vi "DCS_positioningEvan.vi"(8 "error in (no error)":errorcluster, 9 "Data":dbl[](array[numeric])=[0.21428571428571427, 0.8571428571428571, 1.0, 0.21428571428571427, 0.9285714285714285, 0.5, 0.9285714285714285, 0.14285714285714285]) -> (0 "X-Y position":dbl[](array[numeric]), 3 "Normalized Data":dbl[][](array[numeric]))   [LabVIEW 2013]
uses:
  <vilib>/Utility/file.llb/Read From Spreadsheet File (DBL).vi
panel:
  out "Simulated array dimensions":i32[](array[numeric])
  out "output array":dbl[][](array[numeric])=[[0.21428571428571427, 0.8571428571428571, 1.0, 0.21428571428571427, 0.9285714285714285, 0.5, 0.9285714285714285, 0.14285714285714285]]
  out "all rows":dbl[][](array[numeric])
  in  "neg_neg_xy":path=path "C:/Users/Chris/Desktop/DCS(Upgrade)/Simulation data/neg_neg_xy.csv"
  in  "neg_pos_xy":path=path "C:/Users/Chris/Desktop/DCS(Upgrade)/Simulation data/neg_pos_xy.csv"
  in  "pos_pos_xy":path=path "C:/Users/Chris/Desktop/DCS(Upgrade)/Simulation data/pos_pos_xy.csv"
  in  "pos_neg_xy":path=path "C:/Users/Chris/Desktop/DCS(Upgrade)/Simulation data/pos_neg_xy.csv"
  out "min R Sq.":dbl
  in  "pos_neg":path=path "C:/Users/Chris/Desktop/DCS(Upgrade)/Simulation data/pos_neg.csv"
  in  "pos_pos":path=path "C:/Users/Chris/Desktop/DCS(Upgrade)/Simulation data/pos_pos.csv"
  in  "neg_neg":path=path "C:/Users/Chris/Desktop/DCS(Upgrade)/Simulation data/neg_neg.csv"
  in  "neg_pos":path=path "C:/Users/Chris/Desktop/DCS(Upgrade)/Simulation data/neg_pos.csv"
  # "Files"
  # "Information"
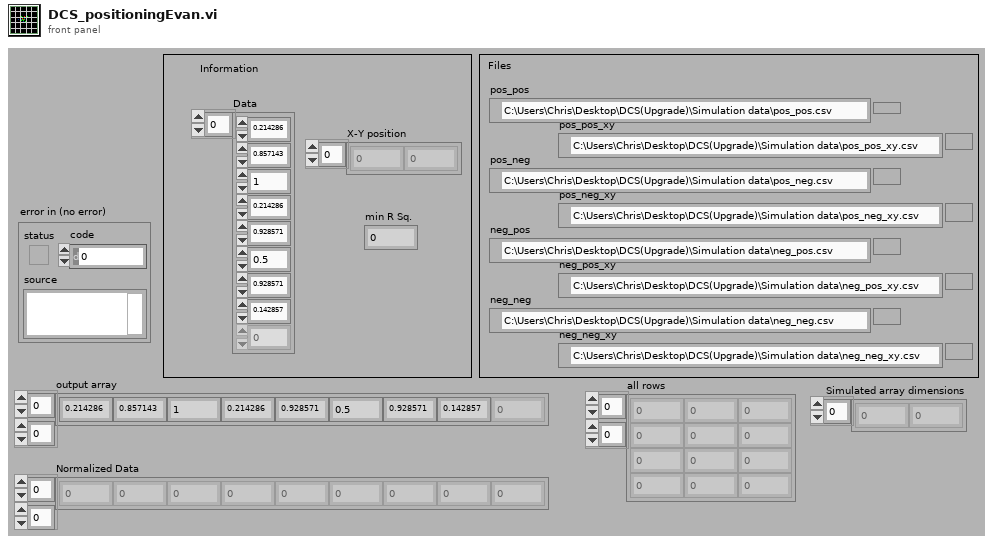
[diagram p1: front panel]
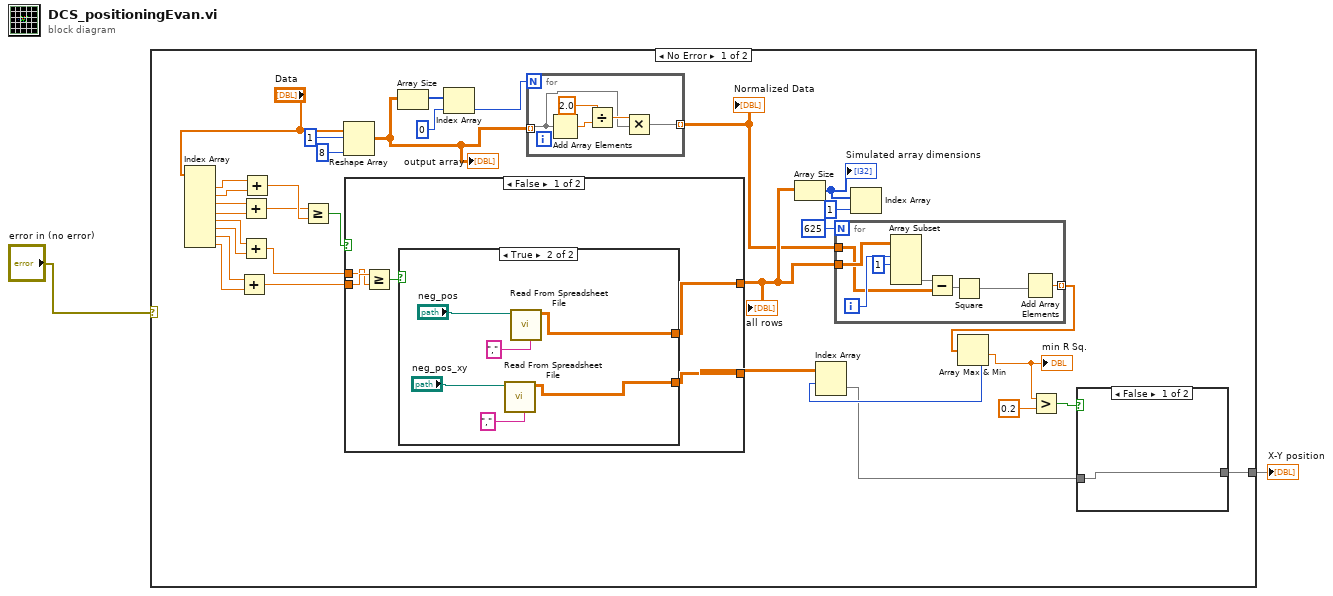
[diagram p0: block diagram]
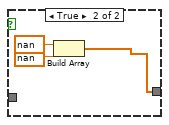
[diagram p2: hidden frame]
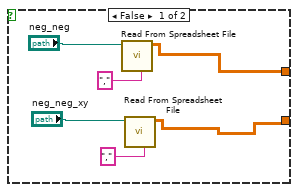
[diagram p3: hidden frame]
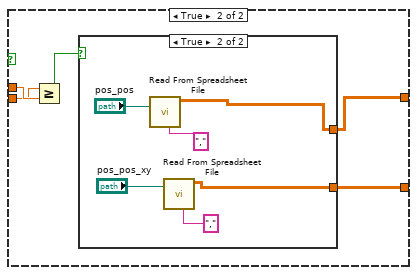
[diagram p4: hidden frame]
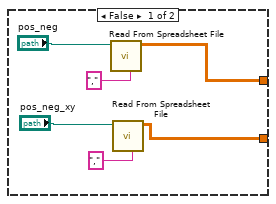
[diagram p5: hidden frame]
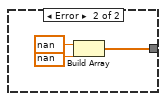
[diagram p6: hidden frame]
diagram:
  n1 = case shown="No Error" "error in (no error)" {
    tunnel: [w9 w87] -> w2
    frame No Error {
      n2 = Index Array(array="Data") -> (element #1=w20:dbl, element #2=w21:dbl, element #3=w22:dbl, element #4=w23:dbl, element #5=w24:dbl, element #6=w25:dbl, element #7=w26:dbl, element #8=w27:dbl)  [unwired: 8 in]
      n3 = Add(x=w26, y=w27) -> (x+y=w31:dbl)
      n4 = Add(x=w22, y=w23) -> (x+y=w33:dbl)
      n5 = Add(x=w24, y=w25) -> (x+y=w32:dbl)
      n6 = Add(x=w20, y=w21) -> (x+y=w34:dbl)
      n7 = Greater Or Equal?(x=w33, y=w34) -> (x >= y?=w35:bool)
      n8 = Reshape Array("Data", 1 ("dimension size"), 8 ("dimension size")) -> (w3:dbl[][])
      "output array" <- w3
      n9 = case shown="False" w35 {
        tunnel: w32 -> [w53 w71]
        tunnel: w31 -> [w54 w70]
        tunnel: [w56 w73] -> w16
        tunnel: [w55 w72] -> w28
        frame False {
          n10 = Greater Or Equal?(x=w54, y=w53) -> (x >= y?=w57:bool)
          n11 = case shown="True" w57 {
            tunnel: [w59 w65] -> w56
            tunnel: [w58 w64] -> w55
            frame False {
              n12 = call-poly <vilib>:"Read From Spreadsheet File.vi"("delimiter (\\t)"="," ("delimiter (\\t)"), "file path (dialog if empty)"="neg_neg") -> ("all rows"=w59:dbl[][])  [unwired: 5 in, 4 out]
              n13 = call-poly <vilib>:"Read From Spreadsheet File.vi"("delimiter (\\t)"="," ("delimiter (\\t)"), "file path (dialog if empty)"="neg_neg_xy") -> ("all rows"=w58:dbl[][])  [unwired: 5 in, 4 out]
            }
            frame True {
              n14 = call-poly <vilib>:"Read From Spreadsheet File.vi"("delimiter (\\t)"="," ("delimiter (\\t)"), "file path (dialog if empty)"="neg_pos_xy") -> ("all rows"=w64:dbl[][])  [unwired: 5 in, 4 out]
              n15 = call-poly <vilib>:"Read From Spreadsheet File.vi"("delimiter (\\t)"="," ("delimiter (\\t)"), "file path (dialog if empty)"="neg_pos") -> ("all rows"=w65:dbl[][])  [unwired: 5 in, 4 out]
            }
          }
        }
        frame True {
          n16 = Greater Or Equal?(x=w70, y=w71) -> (x >= y?=w74:bool)
          n17 = case shown="True" w74 {
            tunnel: [w76 w82] -> w73
            tunnel: [w75 w81] -> w72
            frame False {
              n18 = call-poly <vilib>:"Read From Spreadsheet File.vi"("delimiter (\\t)"="," ("delimiter (\\t)"), "file path (dialog if empty)"="pos_neg") -> ("all rows"=w76:dbl[][])  [unwired: 5 in, 4 out]
              n19 = call-poly <vilib>:"Read From Spreadsheet File.vi"("delimiter (\\t)"="," ("delimiter (\\t)"), "file path (dialog if empty)"="pos_neg_xy") -> ("all rows"=w75:dbl[][])  [unwired: 5 in, 4 out]
            }
            frame True {
              n20 = call-poly <vilib>:"Read From Spreadsheet File.vi"("delimiter (\\t)"="," ("delimiter (\\t)"), "file path (dialog if empty)"="pos_pos") -> ("all rows"=w82:dbl[][])  [unwired: 5 in, 4 out]
              n21 = call-poly <vilib>:"Read From Spreadsheet File.vi"("delimiter (\\t)"="," ("delimiter (\\t)"), "file path (dialog if empty)"="pos_pos_xy") -> ("all rows"=w81:dbl[][])  [unwired: 5 in, 4 out]
            }
          }
        }
      }
      "all rows" <- w16
      n22 = Array Size(array=w3) -> (size(s)=w7:i32[])
      n23 = Index Array(array=w7, index=0) -> (element=w5:i32)
      n24 = for {
        N: w5 -> [_]
        tunnel: w3 -> [w37] mode=indexing
        tunnel: [w36] -> w4 mode=indexing
        n25 = Add Array Elements(numeric array=w37) -> (sum=w40:dbl)
        n26 = Divide(x=2.0, y=w40) -> (x/y=w38:dbl)
        n27 = Multiply(x=w38, y=w37) -> (x*y=w36:dbl[])
      }
      "Normalized Data" <- w4
      n28 = Array Size(array=w16) -> (size(s)=w18:i32[])
      "Simulated array dimensions" <- w18
      n29 = for {
        N: 625 -> [_]
        tunnel: w4 -> [w48]
        tunnel: w16 -> [w49]
        tunnel: [w51] -> w15 mode=indexing
        i -> [w50]
        n30 = Array Subset(array=w49, index (row)=w50, length (row)=1 ("length")) -> (w46:dbl[][])  [unwired: 2 in]
        n31 = Subtract(x=w46, y=w48) -> (x-y=w47:dbl[][])
        n32 = Square(x=w47) -> (x^2=w45:dbl[][])
        n33 = Add Array Elements(numeric array=w45) -> (sum=w51:dbl)
      }
      n34 = Index Array(array=w18, index=1) -> ()  [unwired: 1 out]
      n35 = Array Max & Min(array=w15) -> (min value=w12:dbl, min index (indices)=w14:i32)  [unwired: 2 out]
      "min R Sq." <- w12
      n36 = Index Array(array=w28, index (row)=w14) -> (element=w8:dbl[])  [unwired: 1 in]
      n37 = Greater?(x=w12, y=0.2) -> (0:w10:bool)
      n38 = case shown="False" w10 {
        tunnel: [w41 w42] -> w9
        tunnel: w8 -> [w41 _]
        frame False {
        }
        frame True {
          n39 = Build Array(nan ("element"), nan ("element")) -> (w42:dbl[])
        }
      }
    }
    frame Error {
      n40 = Build Array(nan ("element"), nan ("element")) -> (w87:dbl[])
    }
  }
  "X-Y position" <- w2
